vi "LayerGraphicManipulation.vi"(6 "Ref Color":u32(colorbox), 7 "Radio Buttons":T1=enum."Ellipse", 8 "error in":errorcluster, 9 "New Color":u32(colorbox), 10 "point(x,y)":cluster{"x":i16, "y":i16}, 11 "Layer.lvclass":refnum<class "Layer.lvclass">) -> (0 "error out":errorcluster, 2 "Operation processed?":bool, 3 "Layer.lvclass out":refnum<class "Layer.lvclass">)   [LabVIEW 2021, in "Tools Paint.lvclass"]
uses:
  Class/Tools/Tools Paint.lvclass
  vi.lib/LabVIEW Icon API/lv_icon/Classes/Layer/Layer.lvclass
  Controls/Tools.ctl
  Controls/Pen.ctl
  Controls/Line.ctl
  Controls/Dropper.ctl
  Controls/Fill.ctl
  Controls/IERect.ctl
  Controls/FRect.ctl
  Controls/Circle.ctl
  Controls/FCircle.ctl
  Controls/Rubber.ctl
  Controls/Text.ctl
  Controls/Selection.ctl
  Controls/Move.ctl
  vi.lib/LabVIEW Icon API/lv_icon/lv_icon.lvlib
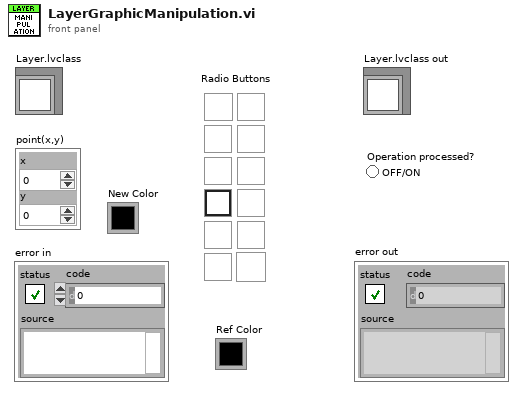
[diagram p1: front panel]
types:
  T1 = typedef "Tools.ctl" = enum32{"Pencil", "Line", "Dropper", "Fill", "Rectangle", "Filled Rectangle", "Ellipse", "Filled Ellipse", "Eraser", "Text", "Select", "Move"}
  T2 = typedef "Layer.ctl" = cluster{"LayerIcon":picture, "LayerName":string, "Opacity":u8, "Visibility?":bool}
  T3 = typedef "LVPoint32TypeDef.ctl" = cluster{"Horizontal":i32, "Vertical":i32}
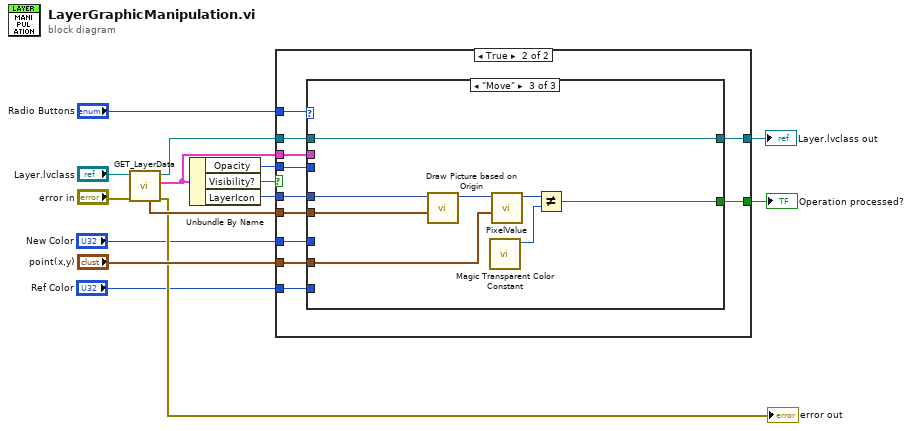
[diagram p0: block diagram]
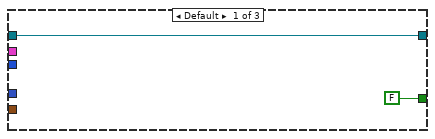
[diagram p3: hidden frame]
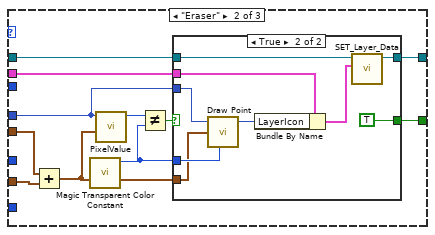
[diagram p4: hidden frame]
diagram:
  n1 = call-dynamic "GET_LayerData.vi"("error in (no error)"="error in", "Layer.lvclass in"="Layer.lvclass") -> ("error out"=→"error out":errorcluster, "Data"=w13:T2, "Layer.lvclass out"=w14:refnum<class "Layer.lvclass">, "Origin"=w10:T3)  [unwired: 6 out]
  n2 = Unbundle By Name(w13) -> ("Opacity"=w7:u8, "Visibility?"=w6:bool, "LayerIcon"=w11:picture)
  n3 = case shown="True" w6 {
    tunnel: w10 -> [_ w26]
    tunnel: w7 -> [_ w20]
    tunnel: w11 -> [_ w27]
    tunnel: "point(x,y)" -> [_ w25]
    tunnel: w13 -> [_ w24]
    tunnel: w14 -> [w16 w23]
    tunnel: [w16 w22] -> w15
    tunnel: "Radio Buttons" -> [_ w21]
    tunnel: [_ w19] -> w3
    tunnel: "New Color" -> [_ w18]
    tunnel: "Ref Color" -> [_ w17]
    frame False {
    }
    frame True {
      n4 = case shown="\"Move\"" w21 {
        tunnel: w27 -> [_ w34 w59]
        tunnel: w26 -> [_ w33 w57]
        tunnel: w25 -> [_ w32 w56]
        tunnel: w24 -> [_ w38 _]
        tunnel: w23 -> [w29 w37 w54]
        tunnel: [w29 w36 w54] -> w22
        tunnel: w20 -> [_ _ _]
        tunnel: [FALSE w35 w53] -> w19
        tunnel: w18 -> [_ _ _]
        tunnel: w17 -> [_ _ _]
        frame Default {
        }
        frame "Eraser" {
          n5 = Add(x=w33, y=w32) -> (x+y=w31:T3)
          n6 = call "Magic Transparent Color Constant.vi"() -> ("Magic transparent color constant"=w30:u32)  [unwired: 11 out]
          n7 = call "PixelValue.vi"("point(x,y)"=w31, "Picture"=w34) -> ("Color"=w40:u32)  [unwired: 9 out]
          n8 = Not Equal?(x=w40, y=w30) -> (x != y?=w39:bool)
          n9 = case shown="True" w39 {
            selector: w39 -> [w41 _]
            tunnel: w30 -> [_ w50]
            tunnel: w31 -> [_ w49]
            tunnel: w38 -> [_ w48]
            tunnel: w34 -> [_ w47]
            tunnel: w37 -> [w42 w45]
            tunnel: [w42 w44] -> w36
            tunnel: [w41 TRUE] -> w35
            frame False {
            }
            frame True {
              n10 = call <vilib>:"Draw Point.vi"("picture"=w47, "point(x,y)"=w49, "color(black)"=w50) -> ("new picture"=w51:picture)  [unwired: 1 in, 5 out]
              n11 = Bundle By Name(cluster=w48, "LayerIcon"=w51) -> (w46:T2)
              n12 = call-dynamic "SET_Layer_Data.vi"("Data"=w46, "Layer.lvclass in"=w45) -> ("Layer.lvclass out"=w44:refnum<class "Layer.lvclass">)  [unwired: 2 in, 7 out]
            }
          }
        }
        frame "Move" {
          n13 = call "Draw Picture based on Origin.vi"("Origin"=w57, "LayerIcon in"=w59) -> ("LayerIcon out"=w55:picture)  [unwired: 1 in, 8 out]
          n14 = call "Magic Transparent Color Constant.vi"() -> ("Magic transparent color constant"=w52:u32)  [unwired: 11 out]
          n15 = call "PixelValue.vi"("point(x,y)"=w56, "Picture"=w55) -> ("Color"=w58:u32)  [unwired: 9 out]
          n16 = Not Equal?(x=w58, y=w52) -> (x != y?=w53:bool)
        }
      }
    }
  }
  "Layer.lvclass out" <- w15
  "Operation processed?" <- w3
